vi "SGUI Set Single Complex Value to String by Label.vi"(0 "label (empty)":string, 1 "value (empty)":cdb=nan+nani, 2 "prefix (empty)":string, 3 "suffix (empty)":string, 5 "format string":string="%.6f", 7 "error in":errorcluster) -> (4 "control ref out":refnum<vi>, 8 "error out":errorcluster)   [LabVIEW 2013, in "varilib.lvlib"]
doc: "This VI formats complex value into 'pretty' string and assigns it to into string control defined by control label (must be registered first by calling 'SGUI Register Controls'). If no value is assigned it will assign empty strings (NaN is considered as no value). It will generate error if control not found or has ivalid type but it ignores input errors (executes anyway)."
uses:
  varilib.lvlib
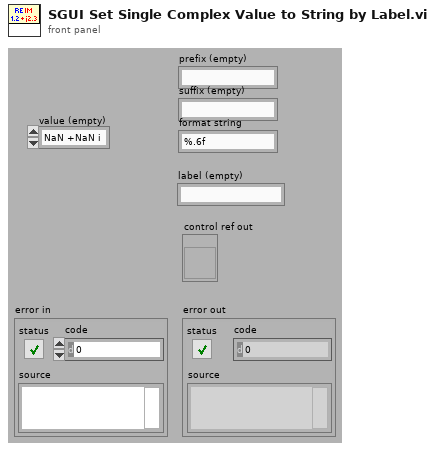
[diagram p1: front panel]
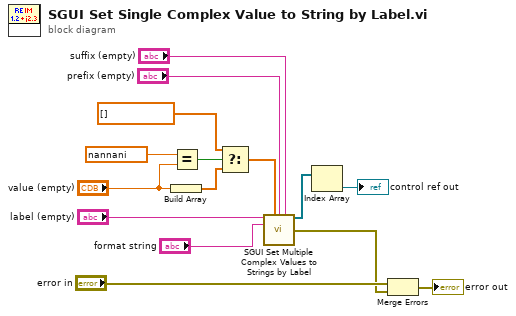
[diagram p0: block diagram]
diagram:
  n1 = Build Array("value (empty)") -> (w10:cdb[])
  n2 = Equal?(x=cdb nan+nani, y="value (empty)") -> (x = y?=w8:bool)
  n3 = Select(t=cdb[] [], s=w8, f=w10) -> (s? t:f=w9:cdb[])
  n4 = call "SGUI Set Multiple Complex Values to Strings by Label.vi"("labels (empty)"="label (empty)", "values (empty)"=w9, "prefix (empty)"="prefix (empty)", "suffix (empty)"="suffix (empty)", "format string"="format string") -> ("assigned control refs"=w6:refnum<vi>[], "error out"=w13:errorcluster)  [unwired: 9 in]
  n5 = Index Array(array=w6) -> (element=→"control ref out":refnum<vi>)  [unwired: 1 in]
  n6 = Merge Errors("error in", w13) -> (→"error out":errorcluster)
